vi "Connection Manager (TDT).vi"(0 "TDT Device Config In":T6, 2 "Parent VI":refnum<vi>, 5 "Properties In":T2, 7 "Endpoint Config":T3[](array[typedef]), 11 "error in (no error)":errorcluster) -> (4 "TDT Device Config Out":T6, 6 "Properties Out":T2, 8 "Canceled?":bool, 15 "error out":errorcluster)   [LabVIEW 2015]
uses:
  PXI DAQ VIs/TDT VIs/Typedefs/TDT-Device Config.ctl
  PXI DAQ VIs/TDT VIs/Typedefs/TDT-Output source.ctl
  PXI DAQ VIs/TDT VIs/Typedefs/TDT-Device ID.ctl
  PXI DAQ VIs/TDT VIs/Typedefs/TDT-Input source.ctl
  Calibration VIs/Endpoint VIs/LV Source/Endpoint-Spec.ctl
  Calibration VIs/Endpoint VIs/LV Source/Endpoint-Modality.ctl
  Calibration VIs/Endpoint VIs/LV Source/Endpoint-Laterality.ctl
  Utility VIs/Buttons/KCheckmarkBoolean 2.ctl
  EPhys/LV Source/Typedefs/EPhys-Hardware Properties.ctl
  D:/Experiment VIs/Misc VIs/Connection Manager/dotNET Source/ConnectionManagerControls/bin/Release/ConnectionManager.dll
  dotNET Source/ConnectionManagerControls/bin/Release/ConnectionManager.dll
panel:
  out "button":bool
  in  "Test Button":bool
  in  "Use kill switch":T1
  in  "Biosemi":T1
  in  "Input":enum16{"Front panel", "RA4LI", "RA16LI"}(ring)
  in  "Connections":refnum<k24>(container)
  out "Image":enum32{"None", "RX6", "RZ5", "RZ6"}(tab)
  in  "Input source":u16(ring) items=["Front panel", "RA4LI", "RA16LI"]
  in  "Run on":u16(ring) items=["RZ5"]
  in  "Cancel":bool
  in  "OK":bool
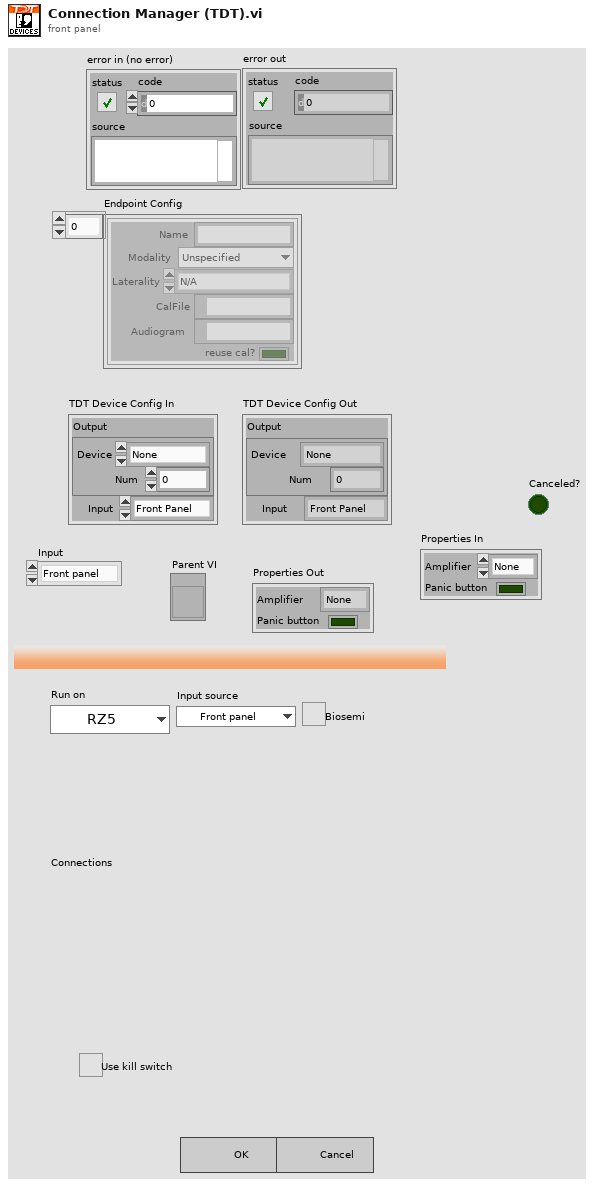
[diagram p1: front panel]
types:
  T1 = typedef "KCheckmarkBoolean 2.ctl" = bool
  T2 = typedef "EPhys-Hardware Properties.ctl" = cluster{"Amplifier":enum16{"None", "Biosemi", "Eclipse", "Eclipse (N.C.)", "Grass"}, "Panic button":bool}
  T3 = typedef "Endpoint-Spec.ctl" = cluster{"Name":string, "Modality":T4, "Laterality":T5, "CalFile":path, "Audiogram":path, "reuse cal?":bool}
  T4 = typedef "Endpoint-Modality.ctl" = enum16{"Unspecified", "Acoustic", "Electric", "Optical"}
  T5 = typedef "Endpoint-Laterality.ctl" = enum16{"N/A", "Right", "Left"}
  T6 = typedef "TDT-Device Config.ctl" = cluster{"Output":T7, "Input":T9}
  T7 = typedef "TDT-Output source.ctl" = cluster{"Device":T8, "Num":i32}
  T8 = typedef "TDT-Device ID.ctl" = enum16{"None", "PA5", "RP2", "RL2", "RA16", "RV8", "RX5", "RX6", "RX7", "RX8", "RZ2", "RZ5", "RZ6"}
  T9 = typedef "TDT-Input source.ctl" = enum16{"Front Panel", "RA4LI", "RA16LI"}
  T10 = enum16{"None", "Biosemi", "Eclipse", "Eclipse (N.C.)", "Grass"}
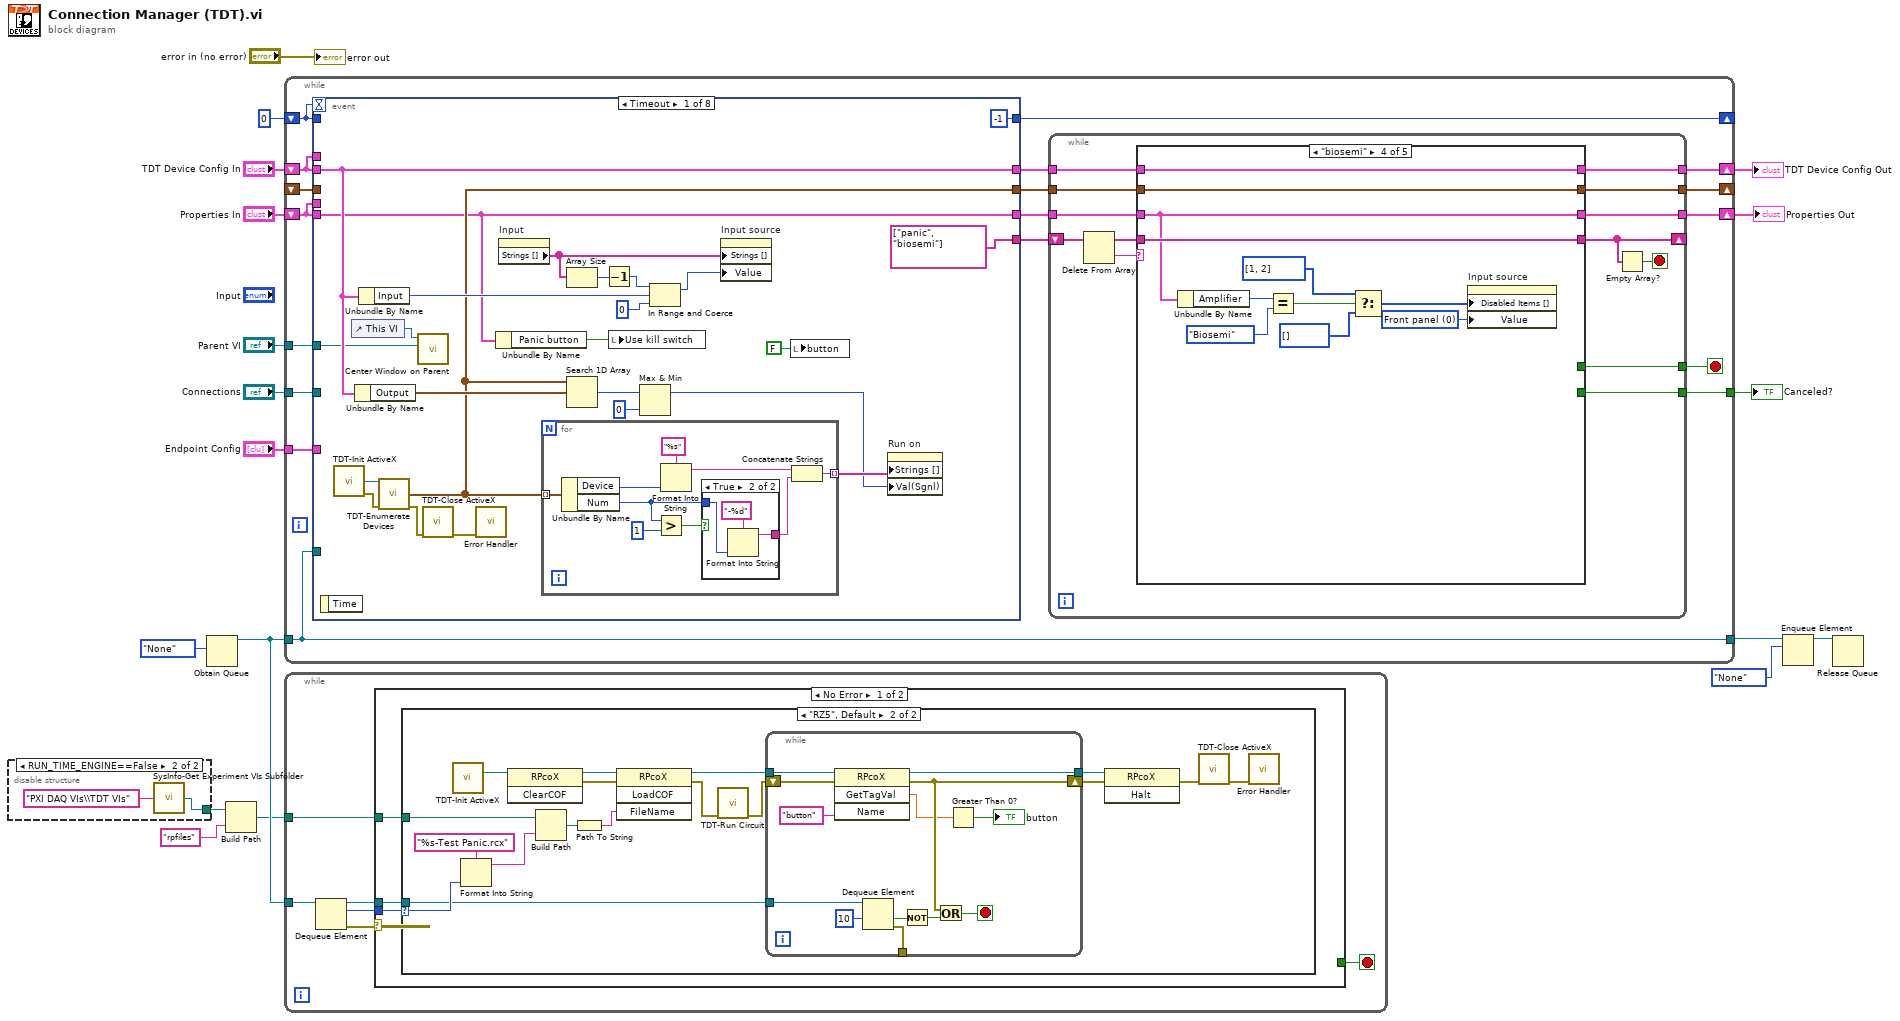
[diagram p0: block diagram]
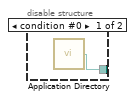
[diagram p2: hidden frame]
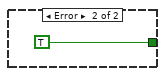
[diagram p4: hidden frame]
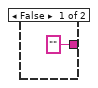
[diagram p5: hidden frame]
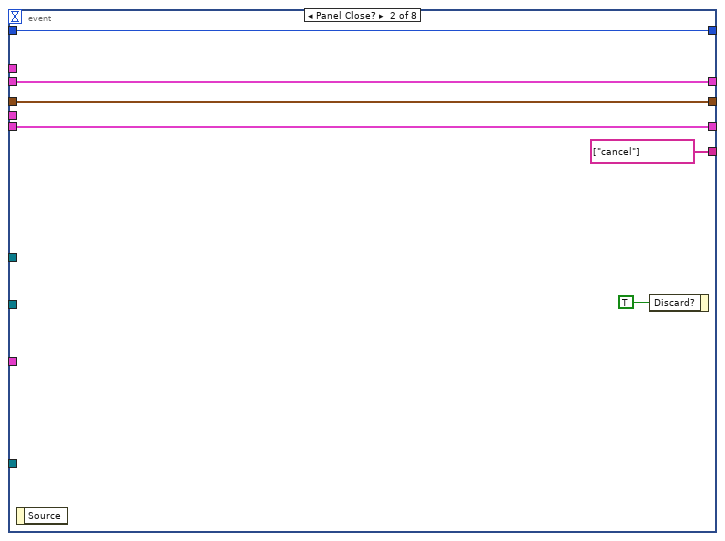
[diagram p6: hidden frame]
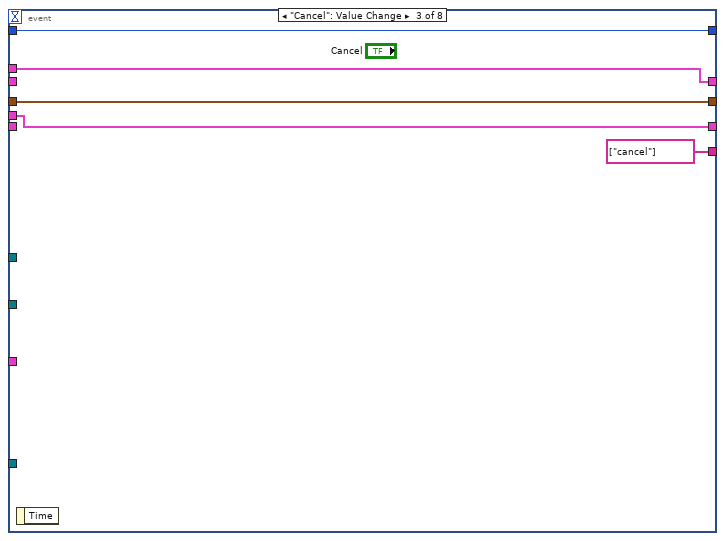
[diagram p7: hidden frame]
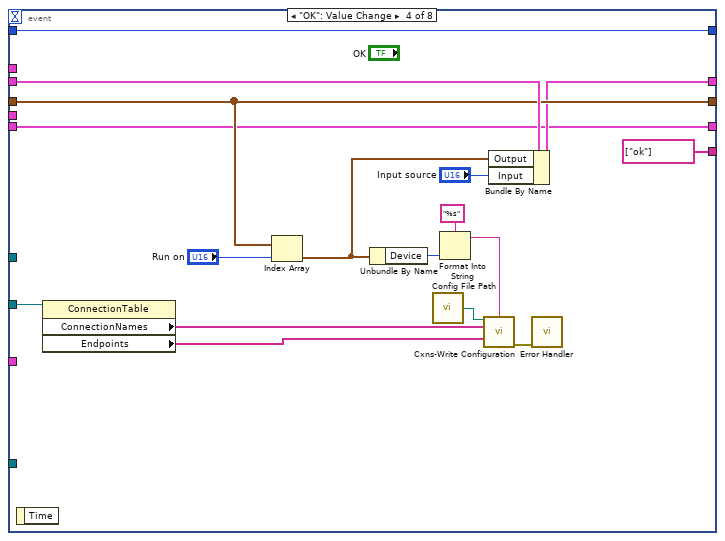
[diagram p8: hidden frame]
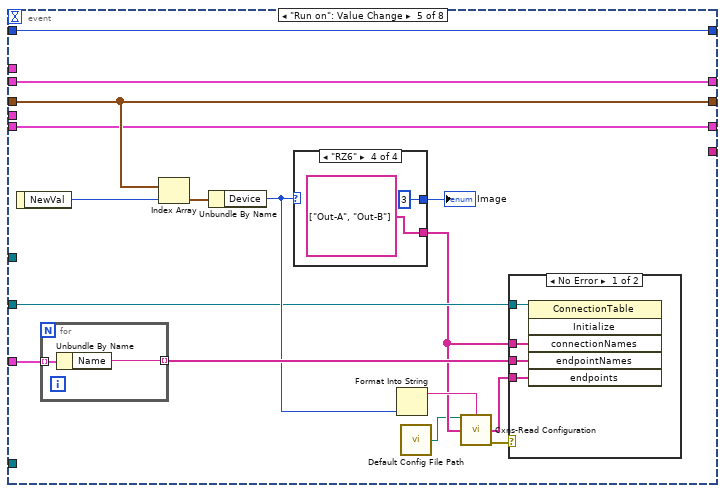
[diagram p9: hidden frame]
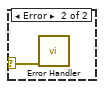
[diagram p10: hidden frame]
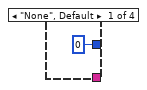
[diagram p11: hidden frame]
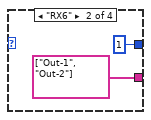
[diagram p12: hidden frame]
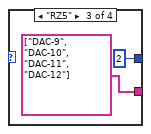
[diagram p13: hidden frame]
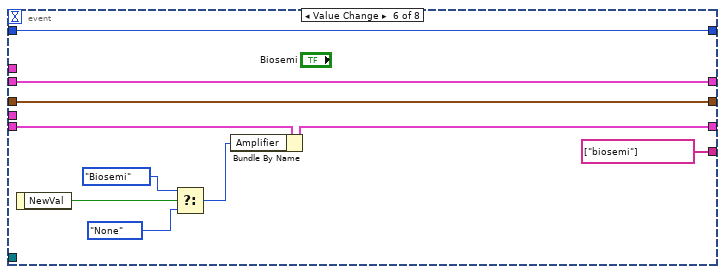
[diagram p14: hidden frame]
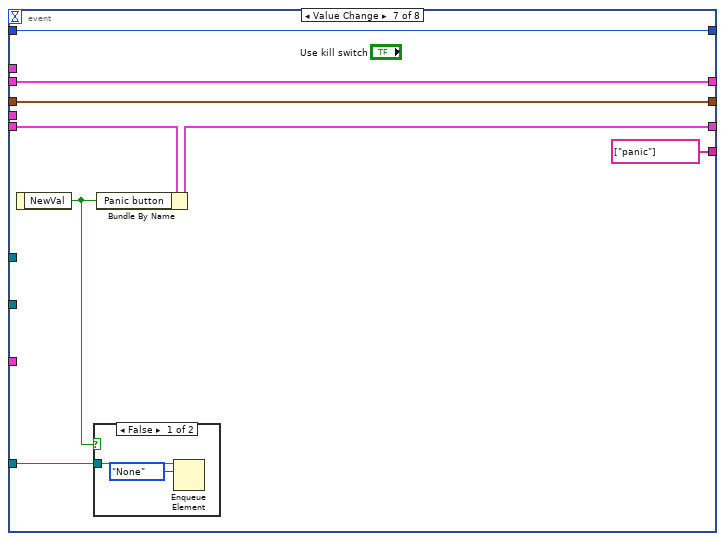
[diagram p15: hidden frame]
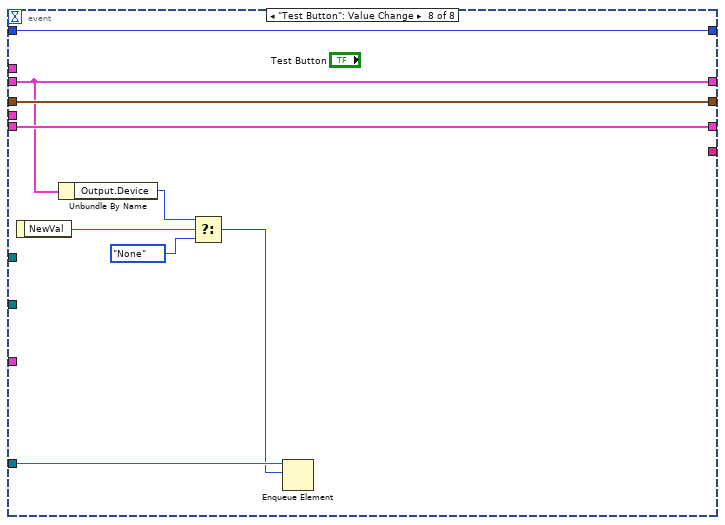
[diagram p17: hidden frame]
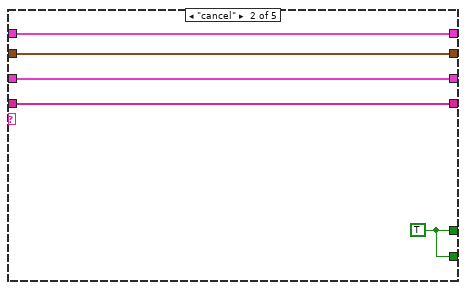
[diagram p19: hidden frame]
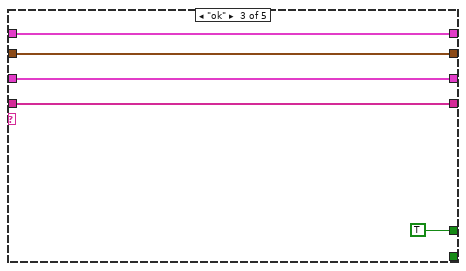
[diagram p20: hidden frame]
diagram:
  n1 = disable-structure shown="RUN_TIME_ENGINE==False" {
    disable-tunnel: [w19 w21] -> w6
    frame condition #0 {
      n2 = call <vilib>:"Application Directory.vi"() -> ("Application Directory"=w19:path)
    }
    frame condition #1 (active) {
      n3 = call "SysInfo-Get Experiment VIs Subfolder.vi"("subfolder"="PXI DAQ VIs\\TDT VIs") -> ("full path"=w21:path)  [unwired: 4 in]
    }
  }
  n4 = Obtain Queue(element data type=TDT-Device_ID."None" ("Output.Device")) -> (queue out=w8:refnum<queue>)  [unwired: 4 in, 2 out]
  n5 = Build Path(base path=w6, name or relative path="rpfiles") -> (appended path=w5:path)
  n6 = while {
    shift-right: [w39] -> _
    shift-left: 0 -> [w37]
    tunnel: [w22] -> w15
    shift-right: [w30] -> w16
    shift-left: "TDT Device Config In" -> [w38]
    shift-right: [w28] -> _
    shift-left: _ -> [w36]
    tunnel: "Connections" -> [w35]
    tunnel: "Endpoint Config" -> [w34]
    tunnel: "Parent VI" -> [w33]
    shift-right: [w26] -> w10
    shift-left: "Properties In" -> [w32]
    tunnel: w8 -> [w23]
    tunnel: [w23] -> w3
    stop <- w24 stop-if-true
    n7 = event shown="[0] Timeout" {
      selector: _ -> [_ _ _ _ _ _ _ _]
      dyn-events: _ -> [_ _ _ _ _ _ _ _]
      timeout: w37 -> [_ _ _ _ _ _ _ _]
      tunnel: [-1 w82 w86 w103 w120 w144 w152 w163] -> w39
      tunnel: w38 -> [w57 w81 _ w104 w119 w143 w151 w160]
      tunnel: [w57 w81 w87 w100 w119 w143 w151 w160] -> w31
      tunnel: w38 -> [_ _ w87 _ _ _ _ _]
      tunnel: w37 -> [_ w82 w86 w103 w120 w144 w152 w163]
      tunnel: [w43 w79 w85 w102 w117 w142 w150 w162] -> w29
      tunnel: w36 -> [_ w79 w85 w102 w117 w142 w150 w162]
      tunnel: w35 -> [_ _ _ w95 w111 _ _ _]
      tunnel: w34 -> [_ _ _ _ w114 _ _ _]
      tunnel: w33 -> [w50 _ _ _ _ _ _ _]
      tunnel: w32 -> [w42 w78 _ w90 w105 w141 w149 w161]
      tunnel: [w42 w78 w84 w90 w105 w140 w148 w161] -> w27
      tunnel: w32 -> [_ _ w84 _ _ _ _ _]
      tunnel: [string[] ["panic", "biosemi"] string[] ["cancel"] string[] ["cancel"] string[] ["ok"] _ string[] ["biosemi"] string[] ["panic"] _] -> w25
      tunnel: w23 -> [_ _ _ _ _ _ w146 w156]
      event Timeout {
        n8 = event-data() -> ()  [unwired: 1 in, 1 out]
        n9 = call "TDT-Init ActiveX.vi"() -> ("ZBUSx"=w48:refnum<k7>, "error out"=w47:errorcluster)  [unwired: 12 in, 2 out]
        n10 = control-ref of="This VI"() -> (w49:refnum<vi>)
        n11 = Unbundle By Name(w57) -> ("Output"=w61:T7)
        n12 = Unbundle By Name(w57) -> ("Input"=w52:T9)
        n13 = call "TDT-Enumerate Devices.vi"("ZBUSx In"=w48, "error in (no error)"=w47) -> ("Devices"=w43:T7[], "error out"=w46:errorcluster)  [unwired: 11 in, 1 out]
        n14 = call "Center Window on Parent.vi"("Parent VI"=w50, "VI in"=w49) -> ()  [unwired: 8 in, 2 out]
        n15 = call "TDT-Close ActiveX.vi"("error in (no error)"=w46) -> ("error out"=w45:errorcluster)  [unwired: 14 in]
        n16 = call "Error Handler.vi"("error in (no error)"=w45) -> ()  [unwired: 13 in, 2 out]
        n17 = Unbundle By Name(w42) -> ("Panic button"=w41:bool)
        n18 = property on="Input" class="Enum (strict)"() -> ("Strings []"=w56:string[])  [unwired: 2 in, 2 out]
        n19 = for {
          tunnel: w43 -> [w72] mode=indexing
          tunnel: [w66] -> w62 mode=indexing
          n20 = Unbundle By Name(w72) -> ("Device"=w64:T8, "Num"=w67:i32)
          n21 = Greater?(x=w67, y=1) -> (0:w68:bool)
          n22 = Format Into String(format string="%s", w64) -> (resulting string=w70:string)  [unwired: 2 in, 1 out]
          n23 = case shown="True" w68 {
            tunnel: w67 -> [_ w75]
            tunnel: ["" w74] -> w65
            frame False {
            }
            frame True {
              n24 = Format Into String(format string="-%d", w75) -> (resulting string=w74:string)  [unwired: 2 in, 1 out]
            }
          }
          n25 = Concatenate Strings(w70, w65) -> (w66:string)
        }
        n26 = Array Size(array=w56) -> (size(s)=w55:i32)
        n27 = Search 1D Array(1D array=w43, element=w61) -> (index of element=w60:i32)  [unwired: 1 in]
        n28 = Decrement(x=w55) -> (x-1=w54:i32)
        n29 = local write "Use kill switch"(w41) -> ()
        n30 = Max & Min(x=w60, y=0) -> (max(x,y)=w58:i32)  [unwired: 1 out]
        n31 = In Range and Coerce(upper limit=w54, x=w52, lower limit=0) -> (coerced(x)=w53:i32)  [unwired: 1 out]
        n32 = property on="Input source" class="Ring (strict)"("Strings []"=w56, "Value"=w53) -> ()  [unwired: 2 in, 2 out]
        n33 = local write "button"(FALSE ("button")) -> ()
        n34 = property on="Run on" class="Ring (strict)"("Strings []"=w62, "Val(Sgnl)"=w58) -> ()  [unwired: 2 in, 2 out]
      }
      event Panel Close? {
        n35 = event-data() -> ()  [unwired: 1 in, 1 out]
        n36 = event-data("Discard?"=TRUE) -> ()  [unwired: 1 in, 1 out]
      }
      event "Cancel": Value Change {
        n37 = event-data() -> ()  [unwired: 1 in, 1 out]
      }
      event "OK": Value Change {
        n38 = event-data() -> ()  [unwired: 1 in, 1 out]
        n39 = property class="ConnectionTable"(reference=w95) -> ("ConnectionNames"=w93:string[], "Endpoints"=w92:string[])  [unwired: 1 in, 2 out]
        n40 = Index Array(array=w102, index="Run on") -> (element=w97:T7)
        n41 = Unbundle By Name(w97) -> ("Device"=w96:T8)
        n42 = call "Config File Path.vi"() -> ("Default config file name"=w89:path)  [unwired: 1 in]
        n43 = Format Into String(format string="%s", w96) -> (resulting string=w94:string)  [unwired: 2 in, 1 out]
        n44 = call "Cxns-Write Configuration.vi"("Connection File Path"=w89, "Section"=w94, "Outputs"=w93, "Endpoints"=w92) -> ("error out"=w91:errorcluster)  [unwired: 11 in]
        n45 = Bundle By Name(cluster=w104, "Output"=w97, "Input"="Input source") -> (w100:T6)
        n46 = call "Error Handler.vi"("error in (no error)"=w91) -> ()  [unwired: 13 in, 2 out]
      }
      event "Run on": Value Change {
        n47 = event-data() -> ("NewVal"=w116:u16)  [unwired: 1 in]
        n48 = for {
          tunnel: w114 -> [w127] mode=indexing
          tunnel: [w126] -> w113 mode=indexing
          n49 = Unbundle By Name(w127) -> ("Name"=w126:string)
        }
        n50 = Index Array(array=w117, index=w116) -> (element=w118:T7)
        n51 = Unbundle By Name(w118) -> ("Device"=w112:T8)
        n52 = case shown="\"RZ6\"" w112 {
          tunnel: [0 1 2 3] -> w115
          tunnel: [_ string[] ["Out-1", "Out-2"] string[] ["DAC-9", "DAC-10", "DAC-11", "DAC-12"] string[] ["Out-A", "Out-B"]] -> w109
          frame "None", Default {
          }
          frame "RX6" {
          }
          frame "RZ5" {
          }
          frame "RZ6" {
          }
        }
        "Image" <- w115
        n53 = Format Into String(w112) -> (resulting string=w110:string)  [unwired: 3 in, 1 out]
        n54 = call "Default Config File Path.vi"() -> ("Default config file name"=w106:path)
        n55 = call "Cxns-Read Configuration.vi"("Connection File Path"=w106, "Section"=w110, "Outputs"=w109) -> ("Endpoints"=w108:string[], "error out"=w107:errorcluster)  [unwired: 11 in]
        n56 = case shown="No Error" w107 {
          selector: w107 -> [_ w125]
          tunnel: w113 -> [w124 _]
          tunnel: w111 -> [w123 _]
          tunnel: w109 -> [w122 _]
          tunnel: w108 -> [w121 _]
          frame No Error {
            n57 = invoke class="ConnectionTable" method="Initialize"(reference=w123, "connectionNames"=w122, "endpointNames"=w124, "endpoints"=w121) -> ()  [unwired: 2 in, 6 out]
          }
          frame Error {
            n58 = call "Error Handler.vi"("error in (no error)"=w125) -> ()  [unwired: 13 in, 2 out]
          }
        }
      }
      event Value Change {
        n59 = event-data() -> ("NewVal"=w137:T1)  [unwired: 1 in]
        n60 = Select(t=T10."Biosemi" ("Amplifier"), s=w137, f=T10."None" ("Amplifier")) -> (s? t:f=w136:T10)
        n61 = Bundle By Name(cluster=w141, "Amplifier"=w136) -> (w140:T2)
      }
      event Value Change {
        n62 = event-data() -> ("NewVal"=w145:T1)  [unwired: 1 in]
        n63 = case shown="False" w145 {
          tunnel: w146 -> [w154 _]
          frame False {
            n64 = Enqueue Element(queue=w154, element=TDT-Device_ID."None") -> ()  [unwired: 2 in, 3 out]
          }
          frame True {
          }
        }
        n65 = Bundle By Name(cluster=w149, "Panic button"=w145) -> (w148:T2)
      }
      event "Test Button": Value Change {
        n66 = event-data() -> ("NewVal"=w159:bool)  [unwired: 1 in]
        n67 = Unbundle By Name(w160) -> ("Output.Device"=w158:T8)
        n68 = Select(t=w158, s=w159, f=TDT-Device_ID."None") -> (s? t:f=w155:T8)
        n69 = Enqueue Element(queue=w156, element=w155) -> ()  [unwired: 2 in, 3 out]
      }
    }
    n70 = while {
      shift-right: [w173] -> _
      shift-left: w25 -> [w176]
      tunnel: w31 -> [w171]
      tunnel: [w170] -> w30
      tunnel: w29 -> [w169]
      tunnel: [w168] -> w28
      tunnel: w27 -> [w167]
      tunnel: [w166] -> w26
      tunnel: [w165] -> w24
      tunnel: [w164] -> w22
      stop <- w172 stop-if-true
      n71 = Delete From Array(array=w176) -> (deleted portion=w174:string, array with subset deleted=w175:string[])  [unwired: 2 in]
      n72 = case shown="\"biosemi\"" w174 {
        tunnel: w175 -> [w180 w185 w190 w201 w207]
        tunnel: [w180 w185 w190 w201 w207] -> w173
        tunnel: w171 -> [w179 w184 w189 w200 w206]
        tunnel: [w179 w184 w189 w200 w206] -> w170
        tunnel: w169 -> [w178 w183 w188 w199 w205]
        tunnel: [w178 w183 w188 w199 w205] -> w168
        tunnel: w167 -> [w177 w182 w187 w196 w204]
        tunnel: [w177 w182 w187 w196 w204] -> w166
        tunnel: [_ w181 TRUE _ _] -> w165
        tunnel: [_ w181 _ _ _] -> w164
        frame "", Default {
        }
        frame "cancel" {
          w181 = TRUE
        }
        frame "ok" {
        }
        frame "biosemi" {
          w192 = u16 0 items=["Front panel", "RA4LI", "RA16LI"] ("Input source")
          n73 = Unbundle By Name(w196) -> ("Amplifier"=w198:T10)
          n74 = Equal?(x=w198, y=T10."Biosemi") -> (x = y?=w191:bool)
          n75 = Select(t=i32[] [1, 2], s=w191, f=i32[] [] ("Disabled Items []")) -> (s? t:f=w194:i32[])
          n76 = property on="Input source" class="Ring (strict)"("Disabled Items []"=w194, "Value"=w192) -> ()  [unwired: 2 in, 2 out]
        }
        frame "panic" {
          n77 = Unbundle By Name(w204) -> ("Panic button"=w203:bool)
          n78 = property on="Test Button" class="Bool (strict)"("Visible"=w203) -> ()  [unwired: 2 in, 2 out]
          n79 = property on="button" class="Bool (strict)"("Visible"=w203, "Value"=FALSE ("button")) -> ()  [unwired: 2 in, 2 out]
        }
      }
      n80 = Empty Array?(array=w173) -> (empty?=w172:bool)
    }
  }
  "TDT Device Config Out" <- w16
  "Canceled?" <- w15
  "Properties Out" <- w10
  n81 = while {
    tunnel: w8 -> [w213]
    tunnel: w5 -> [w210]
    stop <- w211 stop-if-true
    n82 = Dequeue Element(queue=w213) -> (queue out=w208:refnum<queue>, element=w209:T8, error out=w212:errorcluster)  [unwired: 2 in, 1 out]
    n83 = case shown="No Error" w212 {
      tunnel: [_ TRUE] -> w211
      tunnel: w210 -> [w215 _]
      tunnel: w209 -> [w216 _]
      tunnel: w208 -> [w214 _]
      frame No Error {
        n84 = case shown="\"RZ5\", Default" w216 {
          selector: w216 -> [_ w230]
          tunnel: w215 -> [_ w228]
          tunnel: w214 -> [_ w224]
          frame "None" {
          }
          frame "RZ5", Default {
            n85 = call "TDT-Init ActiveX.vi"() -> ("RPcox"=w219:refnum<k7>)  [unwired: 12 in, 3 out]
            n86 = Format Into String(format string="%s-Test Panic.rcx", w230) -> (resulting string=w229:string)  [unwired: 2 in, 1 out]
            n87 = invoke class="RPcoX" method="ClearCOF"(reference=w219) -> (reference out=w233:refnum<k7>, error out=w232:errorcluster)  [unwired: 2 in, 1 out]
            n88 = Build Path(base path=w228, name or relative path=w229) -> (appended path=w227:path)
            n89 = Path To String(path=w227) -> (string=w226:string)
            n90 = invoke class="RPcoX" method="LoadCOF"(reference=w233, error in=w232, "FileName"=w226) -> (reference out=w222:refnum<k7>, error out=w225:errorcluster)  [unwired: 1 in, 2 out]
            n91 = call "TDT-Run Circuit.vi"("error in (no error)"=w225) -> ("error out"=w223:errorcluster)  [unwired: 14 in]
            n92 = while {
              tunnel: w224 -> [w246]
              shift-right: [w238] -> w220
              shift-left: w223 -> [w239]
              tunnel: w222 -> [w240]
              tunnel: [w235] -> w221
              tunnel: [w234] -> _
              stop <- w242 stop-if-true
              n93 = invoke class="RPcoX" method="GetTagVal"(reference=w240, error in=w239, "Name"="button" ("format string")) -> (reference out=w235:refnum<k7>, error out=w238:errorcluster, "GetTagVal"=w237:sgl)  [unwired: 1 in, 1 out]
              n94 = Dequeue Element(queue=w246, timeout in ms (-1)=10) -> (timed out?=w244:bool, error out=w234:errorcluster)  [unwired: 1 in, 2 out]
              n95 = Not(x=w244) -> (.not. x?=w243:bool)
              n96 = Or(x=w238, y=w243) -> (x .or. y?=w242:bool)
              n97 = Greater Than 0?(x=w237) -> (x > 0?=→"button":bool)
            }
            n98 = invoke class="RPcoX" method="Halt"(reference=w221, error in=w220) -> (error out=w218:errorcluster)  [unwired: 1 in, 2 out]
            n99 = call "TDT-Close ActiveX.vi"("error in (no error)"=w218) -> ("error out"=w217:errorcluster)  [unwired: 14 in]
            n100 = call "Error Handler.vi"("error in (no error)"=w217) -> ()  [unwired: 13 in, 2 out]
          }
        }
      }
      frame Error {
      }
    }
  }
  n101 = Enqueue Element(queue=w3, element=TDT-Device_ID."None") -> (queue out=w2:refnum<queue>)  [unwired: 2 in, 2 out]
  n102 = Release Queue(queue=w2) -> ()  [unwired: 2 in, 3 out]
  "error out" <- "error in (no error)"
